vi "Slider Ramp Parameters DAO.vi"(7 "refnum in":T1, 8 "error in (no error)":errorcluster, 9 "SliderRampParameters In":T2={"ramp multiplier"=20.0, "hold multiplier"=3.0, "Delay"=500}, 11 "Persistent DAO Actions":T3) -> (0 "error out":errorcluster, 1 "SliderRampParameters Out":T2={"ramp multiplier"=20.0, "hold multiplier"=3.0, "Delay"=500}, 4 "refnum out":T1)   [LabVIEW 2013]
uses:
  Slider Ramp Parameters.ctl
  Metadata/Persistant DAO Actions.ctl
  <vilib>/Utility/config.llb/Config Data RefNum.ctl
  <vilib>/Utility/config.llb/Write Key (Double).vi
  <vilib>/Utility/config.llb/Write Key (U32).vi
  <vilib>/Utility/config.llb/Read Key (Double).vi
  <vilib>/Utility/config.llb/Read Key (I32).vi
  <vilib>/Utility/config.llb/NI_LVConfig.lvlib
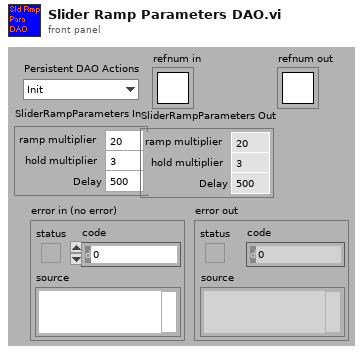
[diagram p1: front panel]
types:
  T1 = typedef "NI_LVConfig.lvlib/Config Data RefNum.ctl" = refnum<k1>
  T2 = typedef "Slider Ramp Parameters.ctl" = cluster{"ramp multiplier":dbl, "hold multiplier":dbl, "Delay":u32}
  T3 = typedef "Persistant DAO Actions.ctl" = enum16{"Init", "Get", "Set", "Load", "Save"}
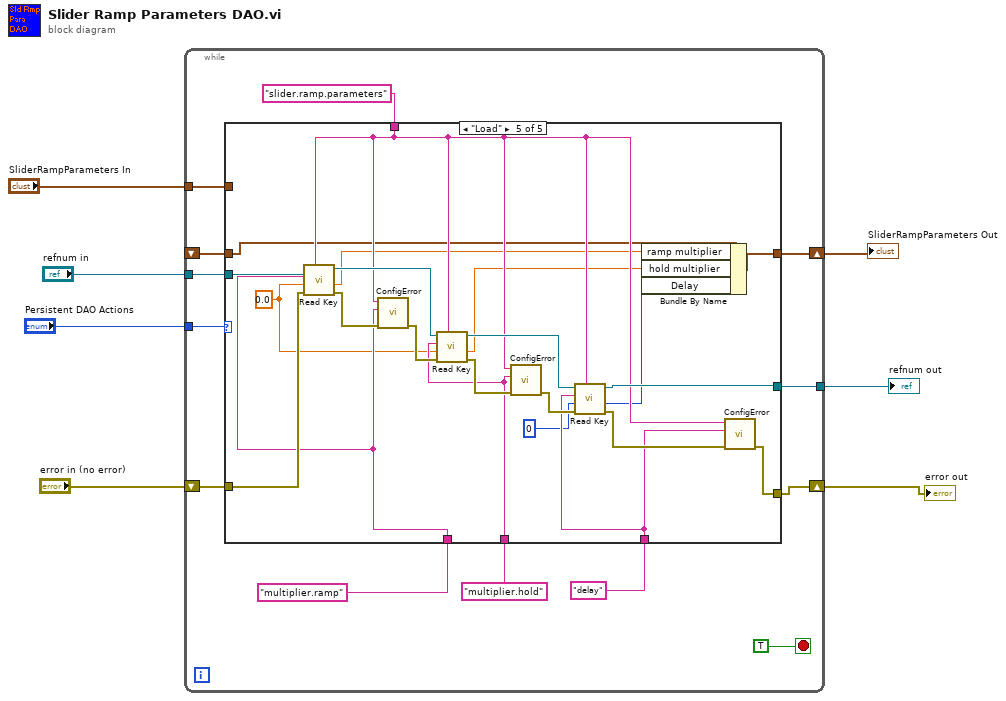
[diagram p0: block diagram]
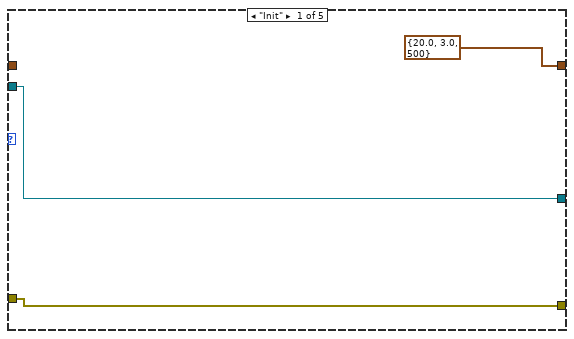
[diagram p2: hidden frame]
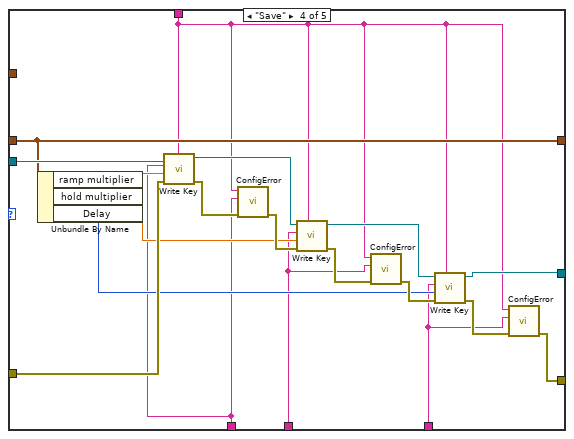
[diagram p5: hidden frame]
diagram:
  n1 = while {
    tunnel: "Persistent DAO Actions" -> [w20]
    tunnel: "SliderRampParameters In" -> [w18]
    shift-right: [w17] -> w5
    shift-left: _ -> [w16]
    shift-right: [w15] -> w4
    shift-left: "error in (no error)" -> [w14]
    tunnel: "refnum in" -> [w13]
    tunnel: [w12] -> w1
    stop <- TRUE stop-if-true
    n2 = case shown="\"Load\"" w20 {
      tunnel: w18 -> [_ _ w29 _ _]
      tunnel: [T2 {"ramp multiplier"=20.0, "hold multiplier"=3.0, "Delay"=500} ("SliderRampParameters In") w26 w29 w37 w52] -> w17
      tunnel: w16 -> [_ w26 _ w37 w53]
      tunnel: [w21 w24 w27 w43 w65] -> w15
      tunnel: w14 -> [w21 w24 w27 w42 w64]
      tunnel: w13 -> [w22 w25 w28 w41 w63]
      tunnel: [w22 w25 w28 w38 w60] -> w12
      tunnel: "slider.ramp.parameters" ("section") -> [_ _ _ w33 w59]
      tunnel: "multiplier.ramp" -> [_ _ _ w32 w58]
      tunnel: "multiplier.hold" -> [_ _ _ w31 w57]
      tunnel: "delay" -> [_ _ _ w30 w56]
      frame "Init" {
      }
      frame "Get" {
      }
      frame "Set" {
      }
      frame "Save" {
        n3 = Unbundle By Name(w37) -> ("ramp multiplier"=w36:dbl, "hold multiplier"=w35:dbl, "Delay"=w34:u32)
        n4 = call-poly <vilib>:"Write Key.vi"("section"=w33, "error in (no error)"=w42, "value"=w36, "key"=w32, "refnum"=w41) -> ("error out"=w48:errorcluster, "refnum out"=w40:T1)  [unwired: 3 in, 2 out]
        n5 = call "ConfigError.vi"("error in (no error)"=w48, "Key"=w32, "Section"=w33) -> ("error out"=w45:errorcluster)  [unwired: 8 out]
        n6 = call-poly <vilib>:"Write Key.vi"("section"=w33, "error in (no error)"=w45, "value"=w35, "key"=w31, "refnum"=w40) -> ("error out"=w47:errorcluster, "refnum out"=w39:T1)  [unwired: 3 in, 2 out]
        n7 = call "ConfigError.vi"("error in (no error)"=w47, "Key"=w31, "Section"=w33) -> ("error out"=w44:errorcluster)  [unwired: 8 out]
        n8 = call-poly <vilib>:"Write Key.vi"("section"=w33, "error in (no error)"=w44, "value"=w34, "key"=w30, "refnum"=w39) -> ("error out"=w46:errorcluster, "refnum out"=w38:T1)  [unwired: 5 out]
        n9 = call "ConfigError.vi"("error in (no error)"=w46, "Key"=w30, "Section"=w33) -> ("error out"=w43:errorcluster)  [unwired: 8 out]
      }
      frame "Load" {
        w55 = 0.0
        n10 = call-poly <vilib>:"Read Key.vi"("section"=w59, "error in (no error)"=w64, "default value"=w55, "key"=w58, "refnum"=w63) -> ("error out"=w70:errorcluster, "value"=w51:dbl, "refnum out"=w62:T1)  [unwired: 4 out]
        n11 = call "ConfigError.vi"("error in (no error)"=w70, "Key"=w58, "Section"=w59) -> ("error out"=w67:errorcluster)  [unwired: 8 out]
        n12 = call-poly <vilib>:"Read Key.vi"("section"=w59, "error in (no error)"=w67, "default value"=w55, "key"=w57, "refnum"=w62) -> ("error out"=w69:errorcluster, "value"=w50:dbl, "refnum out"=w61:T1)  [unwired: 4 out]
        n13 = call "ConfigError.vi"("error in (no error)"=w69, "Key"=w57, "Section"=w59) -> ("error out"=w66:errorcluster)  [unwired: 8 out]
        n14 = call-poly <vilib>:"Read Key.vi"("section"=w59, "error in (no error)"=w66, "default value"=0, "key"=w56, "refnum"=w61) -> ("error out"=w68:errorcluster, "value"=w49:i32, "refnum out"=w60:T1)  [unwired: 4 out]
        n15 = Bundle By Name(cluster=w53, "ramp multiplier"=w51, "hold multiplier"=w50, "Delay"=w49) -> (w52:T2)
        n16 = call "ConfigError.vi"("error in (no error)"=w68, "Key"=w56, "Section"=w59) -> ("error out"=w65:errorcluster)  [unwired: 8 out]
      }
    }
  }
  "SliderRampParameters Out" <- w5
  "error out" <- w4
  "refnum out" <- w1
